vi "about.vi"(8 "服务器信息":T1={"host"="27.154.58.30", "port"=8020, "user"="std", "password"="std23506", "远端地址"="/微站/四代/一体化微型水质监测站.exe"}, 9 "SN输入":string="SN", 10 "站点名称输入":string="站点名称", 11 "应用程序名称输入":string="地表水水质自动监测系统") -> ()   [LabVIEW 2016, in "数据传输系统-03.lvlib" / "update.lvlib"]
uses:
  update.lvlib
  <vilib>/Utility/miscctls.llb/LVPointTypeDef.ctl
panel:
  in  "正式版/测试版":bool
  in  "检查更新":bool
  in  "更新日志":bool
  out "SN":string="SN"
  out "站点名称":string="站点名称"
  out "Version":string="Version 1.0.0"
  out "应用程序名称":string="地表水水质自动监测系统"
  # "关于"
  # "软件名称:"
  # "软件版本:"
  # "站点名称:"
  # "序列号:"
  # "Copyright (c) 2019. All rights reserved."
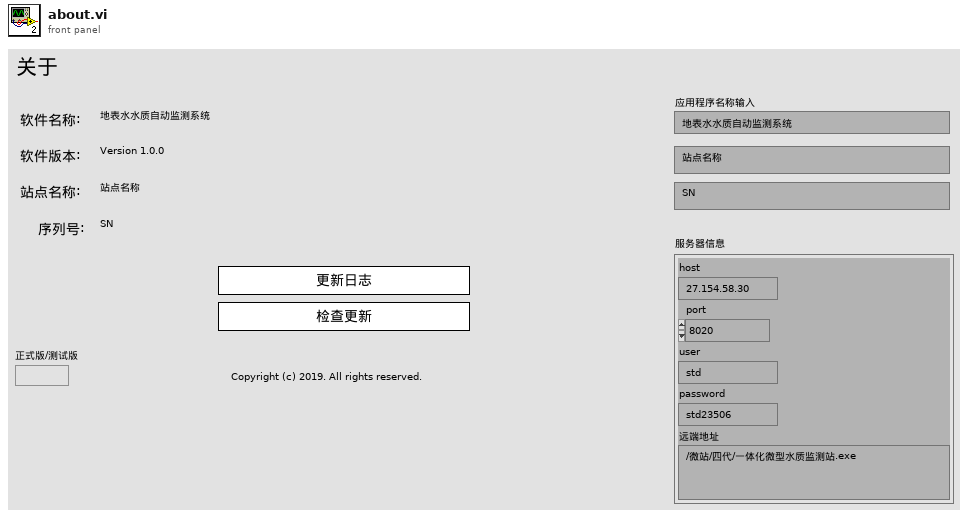
[diagram p1: front panel]
types:
  T1 = cluster{"host":string, "port":u16, "user":string, "password":string, "远端地址":string}
  T2 = typedef "LVPointTypeDef.ctl" = cluster{"Horizontal":i16, "Vertical":i16}
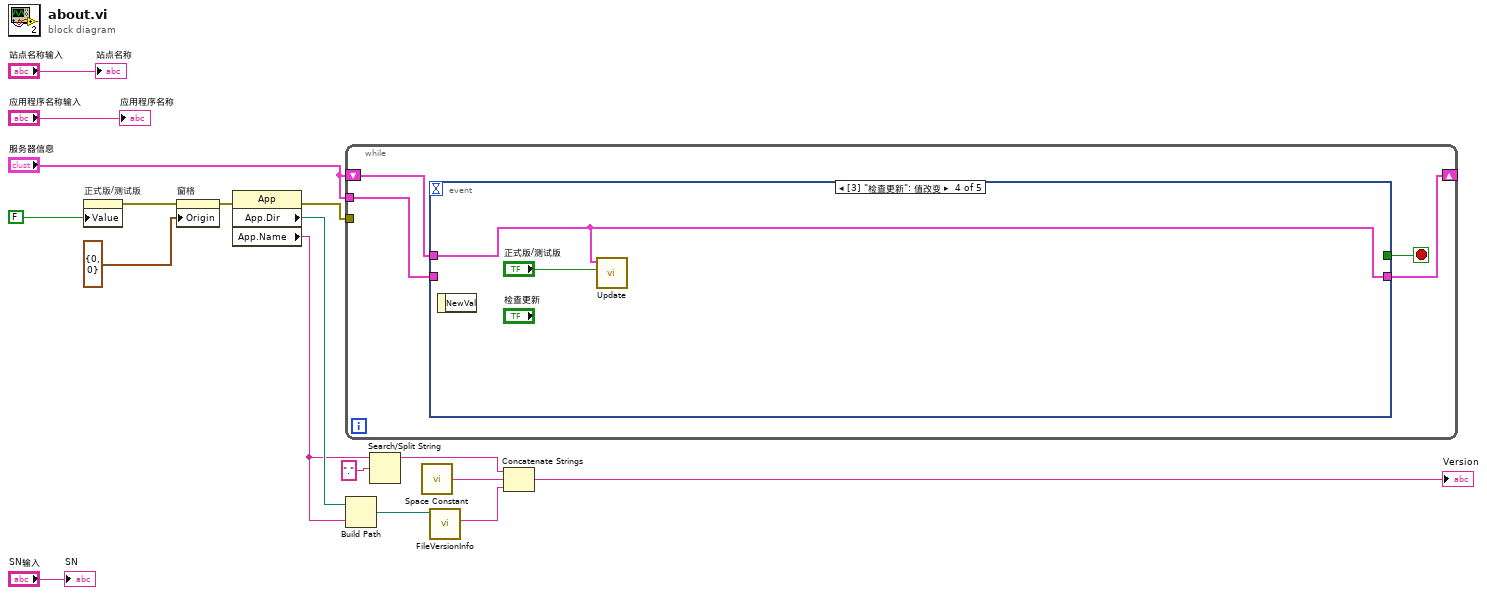
[diagram p0: block diagram]
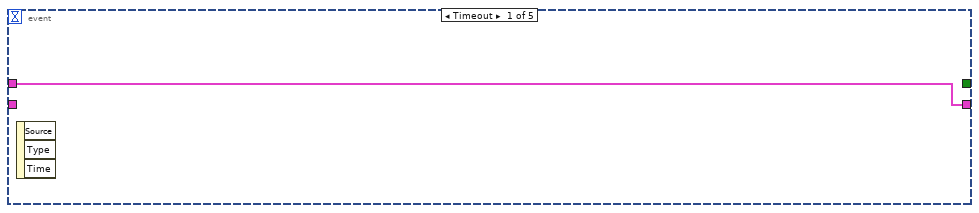
[diagram p2: hidden frame]
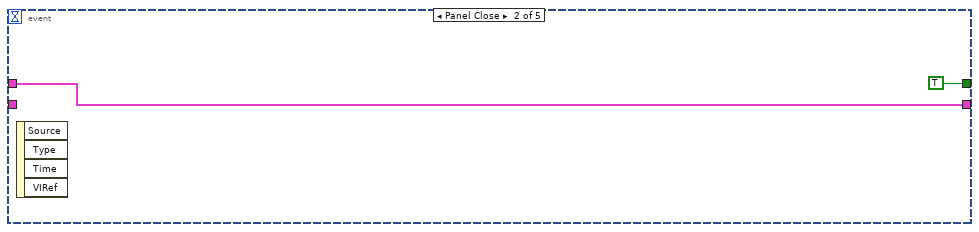
[diagram p3: hidden frame]
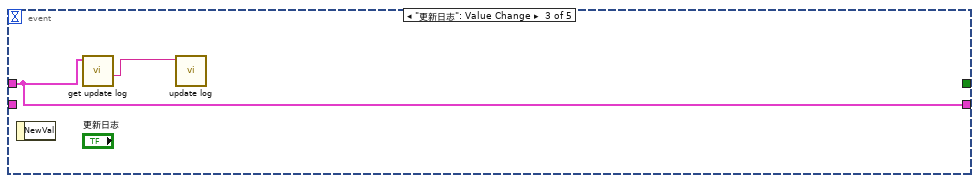
[diagram p4: hidden frame]
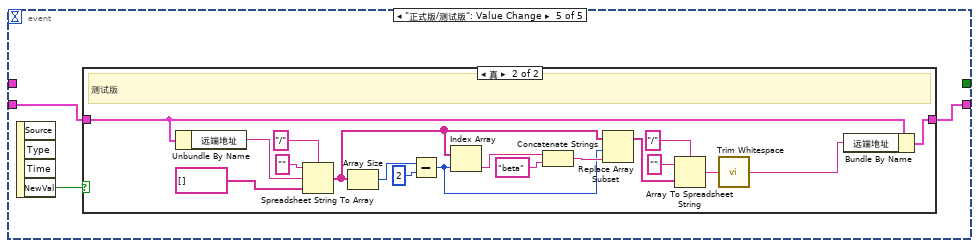
[diagram p5: hidden frame]
diagram:
  n1 = property on="正式版/测试版" class="Bool (严格)"("Value"=FALSE ("正式版/测试版")) -> (error out=w1:errorcluster)  [unwired: 2 in, 1 out]
  n2 = property on="窗格" class="Pane"(error in=w1, "Origin"=T2 {"Horizontal"=0, "Vertical"=0} ("原点")) -> (error out=w4:errorcluster)  [unwired: 1 in, 1 out]
  n3 = property class="App"(error in=w4) -> (error out=w3:errorcluster, "App.Dir"=w16:path, "App.Name"=w15:string)  [unwired: 1 in, 1 out]
  n4 = while {
    shift-right: [w19] -> _
    shift-left: "服务器信息" -> [w20]
    tunnel: "服务器信息" -> [w18]
    tunnel: w3 -> [_]
    stop <- w21 stop-if-true
    n5 = event shown="[3] \"检查更新\": 值改变" {
      selector: _ -> [_ _ _ _ _]
      dyn-events: _ -> [_ _ _ _ _]
      timeout: _ -> [_ _ _ _ _]
      tunnel: [_ TRUE _ _ _] -> w21
      tunnel: w20 -> [w22 w23 w25 w28 _]
      tunnel: [w22 w23 w25 w28 w30] -> w19
      tunnel: w18 -> [_ _ _ _ w29]
      event Timeout {
        n6 = event-data() -> ()  [unwired: 1 in, 3 out]
      }
      event Panel Close {
        n7 = event-data() -> ()  [unwired: 1 in, 4 out]
      }
      event "更新日志": Value Change {
        n8 = event-data() -> ()  [unwired: 1 in, 1 out]
        n9 = call "get update log.vi"("服务器信息"=w25) -> ("部分更新日志"=w26:string)  [unwired: 6 in, 4 out]
        n10 = call "update log.vi"("更新记录"=w26) -> ()  [unwired: 10 in, 1 out]
      }
      event "检查更新": Value Change {
        n11 = event-data() -> ()  [unwired: 1 in, 1 out]
        n12 = call "Update.vi"("测试版？"="正式版/测试版", "服务器信息"=w28) -> ()  [unwired: 10 in]
      }
      event "正式版/测试版": Value Change {
        n13 = event-data() -> ("NewVal"=w31:bool)  [unwired: 1 in, 3 out]
        n14 = case shown="真" w31 {
          tunnel: w29 -> [w32 w50]
          tunnel: [w32 w49] -> w30
          frame False {
            # "默认正式版"
          }
          frame True {
            # "测试版"
            n15 = Unbundle By Name(w50) -> ("远端地址"=w34:string)
            n16 = Spreadsheet String To Array(delimiter (Tab)="/" ("分隔符(Tab)"), format string="", spreadsheet string=w34, array type (2D Dbl)=string[] []) -> (array=w40:string[])
            n17 = Array Size(array=w40) -> (size(s)=w38:i32)
            n18 = Subtract(x=w38, y=2) -> (x-y=w41:i32)
            n19 = Index Array(array=w40, index=w41) -> (element=w42:string)
            n20 = Concatenate Strings(w42, "beta" ("字符串")) -> (w44:string)
            n21 = Replace Array Subset(array=w40, new element=w44, index=w41) -> (w45:string[])
            n22 = Array To Spreadsheet String(delimiter (Tab)="/" ("分隔符(Tab)"), array=w45, 3:"") -> (spreadsheet string=w48:string)
            n23 = call <vilib>:"Trim Whitespace.vi"("string"=w48) -> ("trimmed string"=w33:string)  [unwired: 1 in]
            n24 = Bundle By Name(cluster=w50, "远端地址"=w33) -> (w49:T1)
          }
        }
      }
    }
  }
  n25 = Build Path(base path=w16, name or relative path=w15) -> (appended path=w12:path)
  n26 = Search/Split String(string=w15, search string/char (-)="." ("搜索字符串/字符(-)")) -> (substring before match=w5:string)  [unwired: 1 in, 2 out]
  n27 = call <vilib>:"Space Constant.vi"() -> ("String"=w9:string)
  n28 = call <vilib>:"FileVersionInfo.vi"("Application Path in"=w12) -> ("File Version Info"=w11:string)  [unwired: 7 in, 3 out]
  n29 = Concatenate Strings(w5, w9, w11) -> (→"Version":string)
  "应用程序名称" <- "应用程序名称输入"
  "站点名称" <- "站点名称输入"
  "SN" <- "SN输入"
